vi "_Get Bookmarks for VI.vi"(8 "error in (no error)":errorcluster, 11 "VI":T3) -> (0 "error out":errorcluster, 2 "possible undisplayed bookmarks":bool, 3 "Array of bookmarks":T1)   [LabVIEW 2017, in "CSM_ExampleBrowser.lvlib"]
uses:
  CSM_ExampleBrowser.lvlib
  controls/BMark_VI_Identifier.ctl
  <vilib>/addons/analyzer/_analyzerctrls.llb/VIAnCtl Analysis App Info.ctl
  controls/BMark_Array of Bookmarks.ctl
  controls/BMark_Bookmark Cluster.ctl
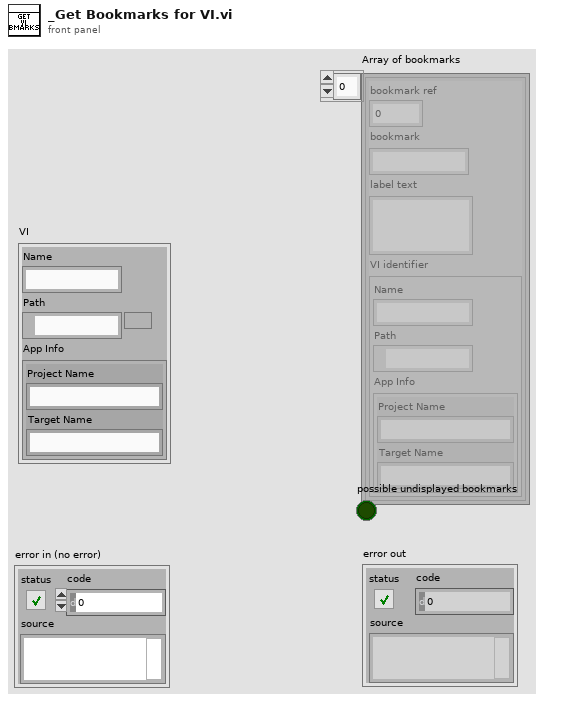
[diagram p1: front panel]
types:
  T1 = typedef "CSM_ExampleBrowser.lvlib/BMark_Array of Bookmarks.ctl" = T2[]
  T2 = typedef "CSM_ExampleBrowser.lvlib/BMark_Bookmark Cluster.ctl" = cluster{"bookmark ref":i32, "bookmark":string, "label text":string, "VI identifier":T3}
  T3 = typedef "CSM_ExampleBrowser.lvlib/BMark_VI_Identifier.ctl" = cluster{"Name":string, "Path":path, "App Info":T4}
  T4 = typedef "VIAnCtl Analysis App Info.ctl" = cluster{"Project Name":string, "Target Name":string}
  T5 = typedef "LVBookmarkInfoTypeDef.ctl" = cluster{"Bookmark Reference":u32, "Bookmark Tag":string, "Label Text":string}[]
  T6 = cluster{"Bookmark Reference":u32, "Bookmark Tag":string, "Label Text":string, "VI":T3}
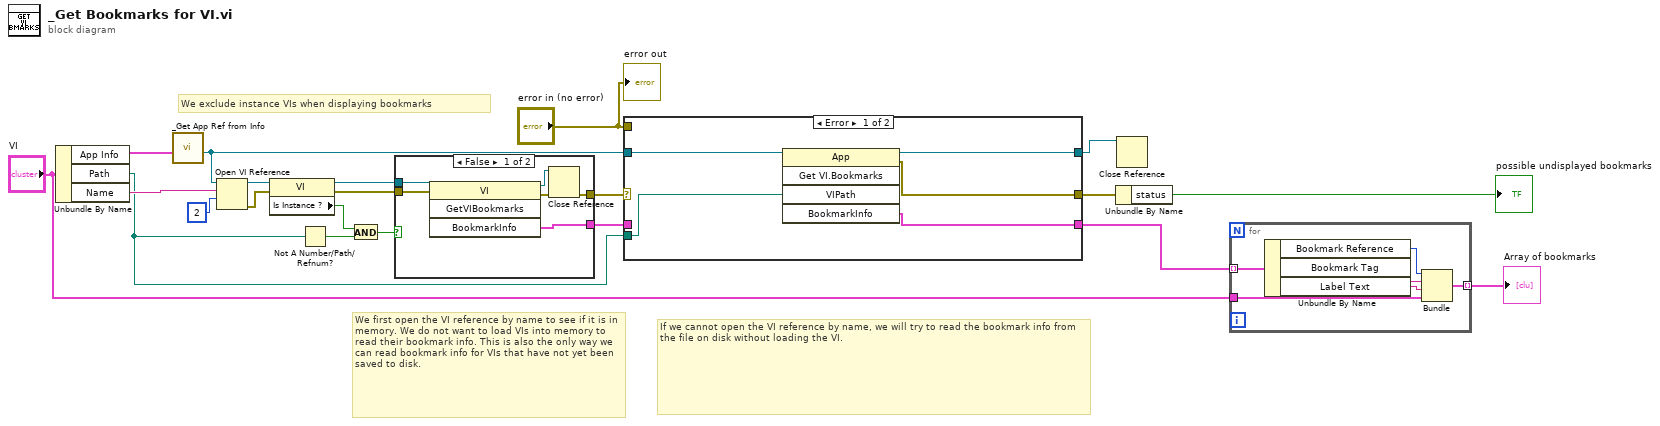
[diagram p0: block diagram]
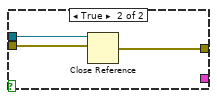
[diagram p2: hidden frame]
diagram:
  # "We exclude instance VIs when displaying bookmarks"
  # "If we cannot open the VI reference by name, we will try to read the bookmark info from the file on disk without loading the VI."
  # "We first open the VI reference by name to see if it is in memory. We do not want to load VIs into memory to read their bookmark info. This is also the only way we can read bookmark info for VIs that have not yet been saved to disk."
  n1 = Unbundle By Name("VI") -> ("App Info"=w14:T4, "Path"=w3:path, "Name"=w16:string)
  n2 = call "_Get App Ref from Info.vi"("Analysis App Info"=w14) -> ("Analysis App ref"=w13:refnum<vi>)  [unwired: 9 in, 1 out]
  n3 = Open VI Reference(application reference (local)=w13, vi path=w16, options=2) -> (vi reference=w8:refnum<vi>, error out=w2:errorcluster)  [unwired: 3 in]
  n4 = property class="VI"(reference=w8, error in=w2) -> (reference out=w7:refnum<vi>, error out=w1:errorcluster, "Is Instance ?"=w6:bool)
  n5 = Not A Number/Path/Refnum?(number/path/refnum=w3) -> (NaN/Path/Refnum?=w5:bool)
  n6 = And(x=w6, y=w5) -> (x .and. y?=w4:bool)
  n7 = case shown="False" w4 {
    tunnel: w1 -> [w27 w29]
    tunnel: [w26 _] -> w17
    tunnel: w7 -> [w25 w30]
    tunnel: [w23 w28] -> w15
    frame False {
      n8 = invoke class="VI" method="GetVIBookmarks"(reference=w25, error in=w27) -> (reference out=w22:refnum<vi>, error out=w24:errorcluster, "BookmarkInfo"=w26:T5)  [unwired: 2 in, 1 out]
      n9 = Close Reference(reference=w22, error in (no error)=w24) -> (error out=w23:errorcluster)
    }
    frame True {
      n10 = Close Reference(reference=w30, error in (no error)=w29) -> (error out=w28:errorcluster)
    }
  }
  n11 = case shown="Error" w15 {
    selector: w15 -> [_ w37]
    tunnel: "error in (no error)" -> [_ _]
    tunnel: [w33 w38] -> w20
    tunnel: w17 -> [_ w38]
    tunnel: w13 -> [w35 w36]
    tunnel: [w34 w37] -> w12
    tunnel: [w32 w36] -> w10
    tunnel: w3 -> [w31 _]
    frame Error {
      n12 = invoke class="App" method="Get VI.Bookmarks"(reference=w35, "VIPath"=w31) -> (reference out=w32:refnum<vi>, error out=w34:errorcluster, "BookmarkInfo"=w33:T5)  [unwired: 3 in, 2 out]
    }
    frame No Error {
    }
  }
  n13 = Unbundle By Name(w12) -> ("status"=→"possible undisplayed bookmarks":bool)
  n14 = Close Reference(reference=w10) -> ()  [unwired: 1 in, 1 out]
  n15 = for {
    tunnel: w20 -> [w44] mode=indexing
    tunnel: "VI" -> [w40]
    tunnel: [w43] -> w19 mode=indexing
    n16 = Unbundle By Name(w44) -> ("Bookmark Reference"=w42:u32, "Bookmark Tag"=w41:string, "Label Text"=w39:string)
    n17 = Bundle("Bookmark Reference"=w42, "Bookmark Tag"=w41, "Label Text"=w39, "VI"=w40) -> (w43:T6)  [unwired: 1 in]
  }
  "Array of bookmarks" <- w19
  "error out" <- "error in (no error)"
